vi "ProfilerTest.vi"() -> ()   [LabVIEW 2014] (continued)
"Velocity"=0.0}, {"Time"=2.6213203435596424, "Velocity"=0.0}, {"Time"=2.6213203435596424, "Velocity"=0.0}, {"Time"=2.6213203435596424, "Velocity"=0.0}, {"Time"=2.6213203435596424, "Velocity"=0.0}, {"Time"=2.6213203435596424, "Velocity"=0.0}, {"Time"=2.6213203435596424, "Velocity"=0.0}, {"Time"=2.6213203435596424, "Velocity"=0.0}, {"Time"=2.6213203435596424, "Velocity"=0.0}, {"Time"=2.6213203435596424, "Velocity"=0.0}, {"Time"=2.6213203435596424, "Velocity"=0.0}, {"Time"=2.6213203435596424, "Velocity"=0.0}, {"Time"=2.6213203435596424, "Velocity"=0.0}, {"Time"=2.6213203435596424, "Velocity"=0.0}, {"Time"=2.6213203435596424, "Velocity"=0.0}, {"Time"=2.6213203435596424, "Velocity"=0.0}, {"Time"=2.6213203435596424, "Velocity"=0.0}, {"Time"=2.6213203435596424, "Velocity"=0.0}, {"Time"=2.6213203435596424, "Velocity"=0.0}, {"Time"=2.6213203435596424, "Velocity"=0.0}, {"Time"=2.6213203435596424, "Velocity"=0.0}, {"Time"=2.6213203435596424, "Velocity"=0.0}, {"Time"=2.6213203435596424, "Velocity"=0.0}, {"Time"=2.6213203435596424, "Velocity"=0.0}, {"Time"=2.6213203435596424, "Velocity"=0.0}, {"Time"=2.6213203435596424, "Velocity"=0.0}, {"Time"=2.6213203435596424, "Velocity"=0.0}, {"Time"=2.6213203435596424, "Velocity"=0.0}, {"Time"=2.6213203435596424, "Velocity"=0.0}, {"Time"=2.6213203435596424, "Velocity"=0.0}, {"Time"=2.6213203435596424, "Velocity"=0.0}, {"Time"=2.6213203435596424, "Velocity"=0.0}, {"Time"=2.6213203435596424, "Velocity"=0.0}, {"Time"=2.6213203435596424, "Velocity"=0.0}, {"Time"=2.6213203435596424, "Velocity"=0.0}, {"Time"=2.6213203435596424, "Velocity"=0.0}, {"Time"=2.6213203435596424, "Velocity"=0.0}, {"Time"=2.6213203435596424, "Velocity"=0.0}, {"Time"=2.6213203435596424, "Velocity"=0.0}, {"Time"=2.6213203435596424, "Velocity"=0.0}, {"Time"=2.6213203435596424, "Velocity"=0.0}, {"Time"=2.6213203435596424, "Velocity"=0.0}, {"Time"=2.6213203435596424, "Velocity"=0.0}, {"Time"=2.6213203435596424, "Velocity"=0.0}, {"Time"=2.6213203435596424, "Velocity"=0.0}, {"Time"=2.6213203435596424, "Velocity"=0.0}, {"Time"=2.6213203435596424, "Velocity"=0.0}, {"Time"=2.6213203435596424, "Velocity"=0.0}, {"Time"=2.6213203435596424, "Velocity"=0.0}, {"Time"=2.6213203435596424, "Velocity"=0.0}, {"Time"=2.6213203435596424, "Velocity"=0.0}, {"Time"=2.6213203435596424, "Velocity"=0.0}, {"Time"=2.6213203435596424, "Velocity"=0.0}, {"Time"=2.6213203435596424, "Velocity"=0.0}, {"Time"=2.6213203435596424, "Velocity"=0.0}, {"Time"=2.6213203435596424, "Velocity"=0.0}, {"Time"=2.6213203435596424, "Velocity"=0.0}, {"Time"=2.6213203435596424, "Velocity"=0.0}, {"Time"=2.6213203435596424, "Velocity"=0.0}, {"Time"=2.6213203435596424, "Velocity"=0.0}, {"Time"=2.6213203435596424, "Velocity"=0.0}, {"Time"=2.6213203435596424, "Velocity"=0.0}, {"Time"=2.6213203435596424, "Velocity"=0.0}, {"Time"=2.6213203435596424, "Velocity"=0.0}, {"Time"=2.6213203435596424, "Velocity"=0.0}, {"Time"=2.6213203435596424, "Velocity"=0.0}, {"Time"=2.6213203435596424, "Velocity"=0.0}, {"Time"=2.6213203435596424, "Velocity"=0.0}, {"Time"=2.6213203435596424, "Velocity"=0.0}, {"Time"=2.6213203435596424, "Velocity"=0.0}, {"Time"=2.6213203435596424, "Velocity"=0.0}, {"Time"=2.6213203435596424, "Velocity"=0.0}, {"Time"=2.6213203435596424, "Velocity"=0.0}, {"Time"=2.6213203435596424, "Velocity"=0.0}, {"Time"=2.6213203435596424, "Velocity"=0.0}, {"Time"=2.6213203435596424, "Velocity"=0.0}, {"Time"=2.6213203435596424, "Velocity"=0.0}, {"Time"=2.6213203435596424, "Velocity"=0.0}, {"Time"=2.6213203435596424, "Velocity"=0.0}, {"Time"=2.6213203435596424, "Velocity"=0.0}, {"Time"=2.6213203435596424, "Velocity"=0.0}, {"Time"=2.6213203435596424, "Velocity"=0.0}, {"Time"=2.6213203435596424, "Velocity"=0.0}, {"Time"=2.6213203435596424, "Velocity"=0.0}, {"Time"=2.6213203435596424, "Velocity"=0.0}, {"Time"=2.6213203435596424, "Velocity"=0.0}, {"Time"=2.6213203435596424, "Velocity"=0.0}, {"Time"=2.6213203435596424, "Velocity"=0.0}, {"Time"=2.6213203435596424, "Velocity"=0.0}, {"Time"=2.6213203435596424, "Velocity"=0.0}, {"Time"=2.6213203435596424, "Velocity"=0.0}, {"Time"=2.6213203435596424, "Velocity"=0.0}, {"Time"=2.6213203435596424, "Velocity"=0.0}, {"Time"=2.6213203435596424, "Velocity"=0.0}, {"Time"=2.6213203435596424, "Velocity"=0.0}, {"Time"=2.6213203435596424, "Velocity"=0.0}, {"Time"=2.6213203435596424, "Velocity"=0.0}, {"Time"=3.179382300521122, "Velocity"=4.887545721840618e-11}, {"Time"=3.182363233638446, "Velocity"=0.004681906750662082}, {"Time"=3.1853442266817455, "Velocity"=0.018707612351687646}, {"Time"=3.1883251621540127, "Velocity"=0.04202122091463451}, {"Time"=3.1913058246256933, "Velocity"=0.0745275081352886}, {"Time"=3.194286771144685, "Velocity"=0.11610430676737167}, {"Time"=3.197267776397191, "Velocity"=0.1665859467999022}, {"Time"=3.2002486616525876, "Velocity"=0.22576990121215637}, {"Time"=3.2032293991934058, "Velocity"=0.2934208962549225}, {"Time"=3.2062103258323984, "Velocity"=0.36927975861350576}, {"Time"=3.2091913664944234, "Velocity"=0.45304642801194395}, {"Time"=3.212172348282649, "Velocity"=0.5443856615355546}, {"Time"=3.215153077010833, "Velocity"=0.6429298808695292}, {"Time"=3.2181341594868247, "Velocity"=0.7483105526778044}, {"Time"=3.2211147839090675, "Velocity"=0.860082815314104}, {"Time"=3.2240958267748936, "Velocity"=0.9778382408534675}, {"Time"=3.2270768318705443, "Velocity"=1.1010952117016748}, {"Time"=3.230057510835584, "Velocity"=1.2293544201841629}, {"Time"=3.2330383537653846, "Velocity"=1.3621303712216255}, {"Time"=3.2360195635020954, "Velocity"=1.4989092093095147}, {"Time"=3.239000371706686, "Velocity"=1.6391158529073055}, {"Time"=3.2419810306914276, "Velocity"=1.7822079438655614}, {"Time"=3.244961997160481, "Velocity"=1.9276428933754883}, {"Time"=3.2479428824398338, "Velocity"=2.074828061328674}, {"Time"=3.2509239694175522, "Velocity"=2.223196577850922}, {"Time"=3.2539048496185483, "Velocity"=2.372142581660095}, {"Time"=3.2568855225487265, "Velocity"=2.5210781729953533}, {"Time"=3.259866572626495, "Velocity"=2.6694447124446374}, {"Time"=3.262847615082643, "Velocity"=2.816637374438716}, {"Time"=3.2658284467512493, "Velocity"=2.962065373403272}, {"Time"=3.2688094528330196, "Velocity"=3.1051735478800238}, {"Time"=3.2717901011492847, "Velocity"=3.245371876903563}, {"Time"=3.2747710323978465, "Velocity"=3.38213728160929}, {"Time"=3.277752022417501, "Velocity"=3.514919121008004}, {"Time"=3.280732985554363, "Velocity"=3.643189467146226}, {"Time"=3.28371363478884, "Velocity"=3.7664305928082165}, {"Time"=3.2866947651209744, "Velocity"=3.8841884916299736}, {"Time"=3.2896756842649046, "Velocity"=3.99597034763491}, {"Time"=3.2926563514365763, "Velocity"=4.101334921685583}, {"Time"=3.2956374727404905, "Velocity"=4.199890633901769}, {"Time"=3.298618474379659, "Velocity"=4.291228403037818}, {"Time"=3.3015991540634593, "Velocity"=4.374983206384261}, {"Time"=3.304580116567556, "Velocity"=4.450841624260995}, {"Time"=3.30756083324709, "Velocity"=4.518490720524196}, {"Time"=3.3105420315563414, "Velocity"=4.577678998720427}, {"Time"=3.3135226724363, "Velocity"=4.628152609214704}, {"Time"=3.3165035991129286, "Velocity"=4.669727810948797}, {"Time"=3.319484620882282, "Velocity"=4.702236153213752}, {"Time"=3.322465509870618, "Velocity"=4.725547028669758}, {"Time"=3.3254465442327077, "Velocity"=4.739570548002267}, {"Time"=3.3284274714794138, "Velocity"=4.744249999882863}, {"Time"=3.3314083274309976, "Velocity"=4.739567811399099}, {"Time"=3.334389068020796, "Velocity"=4.725543407232389}, {"Time"=3.33736999085439, "Velocity"=4.702230421822115}, {"Time"=3.3403510145205813, "Velocity"=4.66972018065884}, {"Time"=3.343331845683909, "Velocity"=4.62814460377215}, {"Time"=3.3463127213565964, "Velocity"=4.577665140474008}, {"Time"=3.34929362108914, "Velocity"=4.518481048135488}, {"Time"=3.352274603067483, "Velocity"=4.450824289890841}, {"Time"=3.355255244905396, "Velocity"=4.3749725174933545}, {"Time"=3.358236366672093, "Velocity"=4.291203685185305}, {"Time"=3.3612170640143364, "Velocity"=4.19987352692686}, {"Time"=3.364197991665377, "Velocity"=4.101323178207656}, {"Time"=3.3671788958736792, "Velocity"=3.995949202532643}, {"Time"=3.370160002773235, "Velocity"=3.884158907986906}, {"Time"=3.373140697172389, "Velocity"=3.7664171646877844}, {"Time"=3.3761216862348933, "Velocity"=3.6431611066430656}, {"Time"=3.3791025119642133, "Velocity"=3.5148957069092033}, {"Time"=3.3820835823865347, "Velocity"=3.3821094679110097}, {"Time"=3.385064249730449, "Velocity"=3.245355564920387}, {"Time"=3.388045261129964, "Velocity"=3.10513959694406}, {"Time"=3.391026157018598, "Velocity"=2.962036133344201}, {"Time"=3.3940071550211357, "Velocity"=2.8165995512860045}, {"Time"=3.39698801785475, "Velocity"=2.6694154211857586}, {"Time"=3.399968948751446, "Velocity"=2.521054654482557}, {"Time"=3.4029497889706777, "Velocity"=2.372110652197633}, {"Time"=3.4059306352291676, "Velocity"=2.2231664051676723}, {"Time"=3.408911705934191, "Velocity"=2.07479887461014}, {"Time"=3.4118924656591023, "Velocity"=1.92762016228879}, {"Time"=3.414873470780533, "Velocity"=1.782183658015315}, {"Time"=3.4178541398265025, "Velocity"=1.6390915280380804}, {"Time"=3.4208351340590917, "Velocity"=1.4988767804771501}, {"Time"=3.4238160119268155, "Velocity"=1.362113826815595}, {"Time"=3.4267971471880583, "Velocity"=1.229325588696039}, {"Time"=3.4297779598240212, "Velocity"=1.1010617891916208}, {"Time"=3.4327588330093084, "Velocity"=0.9778115520210151}, {"Time"=3.435739589972038, "Velocity"=0.8600684112964558}, {"Time"=3.4387207610191526, "Velocity"=0.7482770016761722}, {"Time"=3.441701442053643, "Velocity"=0.6429121146564376}, {"Time"=3.4446823370875865, "Velocity"=0.544363817902734}, {"Time"=3.4476634251575002, "Velocity"=0.45302316196243675}, {"Time"=3.450644092312822, "Velocity"=0.3692685559349724}, {"Time"=3.4536252188140226, "Velocity"=0.29340600994766153}, {"Time"=3.456605936904525, "Velocity"=0.22575715851294909}, {"Time"=3.4595868836619856, "Velocity"=0.16657379756771834}, {"Time"=3.4625677175232754, "Velocity"=0.11609675641697091}, {"Time"=3.4655485614792525, "Velocity"=0.07452270710143796}, {"Time"=3.4685295280726667, "Velocity"=0.04201475404893379}, {"Time"=3.471510361955229, "Velocity"=0.018703923478933956}, {"Time"=3.474491413705976, "Velocity"=0.004679874386484596}, {"Time"=3.477472452833142, "Velocity"=1.0614160298802687e-10}, {"Time"=3.82842712474619, "Velocity"=0.0}, {"Time"=3.82842712474619, "Velocity"=0.0}, {"Time"=3.82842712474619, "Velocity"=0.0}, {"Time"=3.82842712474619, "Velocity"=0.0}, {"Time"=3.82842712474619, "Velocity"=0.0}, {"Time"=3.82842712474619, "Velocity"=0.0}, {"Time"=3.82842712474619, "Velocity"=0.0}, {"Time"=3.82842712474619, "Velocity"=0.0}, {"Time"=3.82842712474619, "Velocity"=0.0}, {"Time"=3.82842712474619, "Velocity"=0.0}, {"Time"=3.82842712474619, "Velocity"=0.0}, {"Time"=3.82842712474619, "Velocity"=0.0}, {"Time"=3.82842712474619, "Velocity"=0.0}, {"Time"=3.82842712474619, "Velocity"=0.0}, {"Time"=3.82842712474619, "Velocity"=0.0}, {"Time"=3.82842712474619, "Velocity"=0.0}, {"Time"=3.82842712474619, "Velocity"=0.0}, {"Time"=3.82842712474619, "Velocity"=0.0}, {"Time"=3.82842712474619, "Velocity"=0.0}, {"Time"=3.82842712474619, "Velocity"=0.0}, {"Time"=3.82842712474619, "Velocity"=0.0}, {"Time"=3.82842712474619, "Velocity"=0.0}, {"Time"=3.82842712474619, "Velocity"=0.0}, {"Time"=3.82842712474619, "Velocity"=0.0}, {"Time"=3.82842712474619, "Velocity"=0.0}, {"Time"=3.82842712474619, "Velocity"=0.0}, {"Time"=3.82842712474619, "Velocity"=0.0}, {"Time"=3.82842712474619, "Velocity"=0.0}, {"Time"=3.82842712474619, "Velocity"=0.0}, {"Time"=3.82842712474619, "Velocity"=0.0}, {"Time"=3.82842712474619, "Velocity"=0.0}, {"Time"=3.82842712474619, "Velocity"=0.0}, {"Time"=3.82842712474619, "Velocity"=0.0}, {"Time"=3.82842712474619, "Velocity"=0.0}, {"Time"=3.82842712474619, "Velocity"=0.0}, {"Time"=3.82842712474619, "Velocity"=0.0}, {"Time"=3.82842712474619, "Velocity"=0.0}, {"Time"=3.82842712474619, "Velocity"=0.0}, {"Time"=3.82842712474619, "Velocity"=0.0}, {"Time"=3.82842712474619, "Velocity"=0.0}, {"Time"=3.82842712474619, "Velocity"=0.0}, {"Time"=3.82842712474619, "Velocity"=0.0}, {"Time"=3.82842712474619, "Velocity"=0.0}, {"Time"=3.82842712474619, "Velocity"=0.0}, {"Time"=3.82842712474619, "Velocity"=0.0}, {"Time"=3.82842712474619, "Velocity"=0.0}, {"Time"=3.82842712474619, "Velocity"=0.0}, {"Time"=3.82842712474619, "Velocity"=0.0}, {"Time"=3.82842712474619, "Velocity"=0.0}, {"Time"=3.82842712474619, "Velocity"=0.0}, {"Time"=3.82842712474619, "Velocity"=0.0}, {"Time"=3.82842712474619, "Velocity"=0.0}, {"Time"=3.82842712474619, "Velocity"=0.0}, {"Time"=3.82842712474619, "Velocity"=0.0}, {"Time"=3.82842712474619, "Velocity"=0.0}, {"Time"=3.82842712474619, "Velocity"=0.0}, {"Time"=3.82842712474619, "Velocity"=0.0}, {"Time"=3.82842712474619, "Velocity"=0.0}, {"Time"=3.82842712474619, "Velocity"=0.0}, {"Time"=3.82842712474619, "Velocity"=0.0}, {"Time"=3.82842712474619, "Velocity"=0.0}, {"Time"=3.82842712474619, "Velocity"=0.0}, {"Time"=3.82842712474619, "Velocity"=0.0}, {"Time"=3.82842712474619, "Velocity"=0.0}, {"Time"=3.82842712474619, "Velocity"=0.0}, {"Time"=3.82842712474619, "Velocity"=0.0}, {"Time"=3.82842712474619, "Velocity"=0.0}, {"Time"=3.82842712474619, "Velocity"=0.0}, {"Time"=3.82842712474619, "Velocity"=0.0}, {"Time"=3.82842712474619, "Velocity"=0.0}, {"Time"=3.82842712474619, "Velocity"=0.0}, {"Time"=3.82842712474619, "Velocity"=0.0}, {"Time"=3.82842712474619, "Velocity"=0.0}, {"Time"=3.82842712474619, "Velocity"=0.0}, {"Time"=3.82842712474619, "Velocity"=0.0}, {"Time"=3.82842712474619, "Velocity"=0.0}, {"Time"=3.82842712474619, "Velocity"=0.0}, {"Time"=3.82842712474619, "Velocity"=0.0}, {"Time"=3.82842712474619, "Velocity"=0.0}, {"Time"=3.82842712474619, "Velocity"=0.0}, {"Time"=3.82842712474619, "Velocity"=0.0}, {"Time"=3.82842712474619, "Velocity"=0.0}, {"Time"=3.82842712474619, "Velocity"=0.0}, {"Time"=3.82842712474619, "Velocity"=0.0}, {"Time"=3.82842712474619, "Velocity"=0.0}, {"Time"=3.82842712474619, "Velocity"=0.0}, {"Time"=3.82842712474619, "Velocity"=0.0}, {"Time"=3.82842712474619, "Velocity"=0.0}, {"Time"=3.82842712474619, "Velocity"=0.0}, {"Time"=3.82842712474619, "Velocity"=0.0}, {"Time"=3.82842712474619, "Velocity"=0.0}, {"Time"=3.82842712474619, "Velocity"=0.0}, {"Time"=3.82842712474619, "Velocity"=0.0}, {"Time"=3.82842712474619, "Velocity"=0.0}, {"Time"=3.82842712474619, "Velocity"=0.0}, {"Time"=3.82842712474619, "Velocity"=0.0}, {"Time"=3.82842712474619, "Velocity"=0.0}, {"Time"=3.82842712474619, "Velocity"=0.0}, {"Time"=3.82842712474619, "Velocity"=0.0}, {"Time"=3.82842712474619, "Velocity"=0.0}, {"Time"=3.82842712474619, "Velocity"=0.0}]}, ...(2 in all)]
  out "XY Graph":T5(graph)=[{"XY Graph"=[{"X"=0.0, "Y"=0.0}, {"X"=0.0, "Y"=0.5}, {"X"=0.5, "Y"=1.0}, {"X"=1.0, "Y"=0.5}, {"X"=0.5, "Y"=0.0}, {"X"=0.0, "Y"=0.5}]}, {"XY Graph"=[{"X"=0.0, "Y"=0.029735763271532455}, {"X"=0.0, "Y"=0.03498550646188265}, {"X"=0.0, "Y"=0.04073166444158789}, {"X"=0.0, "Y"=0.046965098069385154}, {"X"=0.0, "Y"=0.053670825690082614}, {"X"=0.0, "Y"=0.06082839203263177}, {"X"=0.0, "Y"=0.06841237188678788}, {"X"=0.0, "Y"=0.0763929961561675}, {"X"=0.0, "Y"=0.0847368848721995}, {"X"=0.0, "Y"=0.09340786911973305}, {"X"=0.0, "Y"=0.10236788163576621}, {"X"=0.0, "Y"=0.11157789415179944}, {"X"=0.0, "Y"=0.12099887839933296}, {"X"=0.0, "Y"=0.1305927671153649}, {"X"=0.0, "Y"=0.14032339138474453}, {"X"=0.0, "Y"=0.15015737123890066}, {"X"=0.0, "Y"=0.16006493758144982}, {"X"=0.0, "Y"=0.1700206652021473}, {"X"=0.0, "Y"=0.18000409882994453}, {"X"=0.0, "Y"=0.19000025680964983}, {"X"=0.0, "Y"=0.20000000000000004}, {"X"=0.0, "Y"=0.21000000000000005}, {"X"=0.0, "Y"=0.22000000000000006}, {"X"=0.0, "Y"=0.23000000000000007}, {"X"=0.0, "Y"=0.24000000000000007}, {"X"=0.0, "Y"=0.25000000000000006}, {"X"=0.0, "Y"=0.26000000000000006}, {"X"=0.0, "Y"=0.2700000000000001}, {"X"=0.0, "Y"=0.2800000000000001}, {"X"=0.0, "Y"=0.2900000000000001}, {"X"=0.0, "Y"=0.3000000000000001}, {"X"=0.0, "Y"=0.3100000000000001}, {"X"=0.0, "Y"=0.3200000000000001}, {"X"=0.0, "Y"=0.3300000000000001}, {"X"=0.0, "Y"=0.34000000000000014}, {"X"=3.652435472123461e-11, "Y"=0.35000000000000014}, {"X"=2.9356280516375233e-07, "Y"=0.36000000000000015}, {"X"=5.746236574666157e-06, "Y"=0.37000000000000016}, {"X"=3.086411351601627e-05, "Y"=0.38000000000000017}, {"X"=9.978288886692112e-05, "Y"=0.3900000000000002}, {"X"=0.00024519954102164955, "Y"=0.3999999811877839}, {"X"=0.0005069250135350944, "Y"=0.40999991604546854}, {"X"=0.00093012200045119, "Y"=0.41999565182389387}, {"X"=0.0015633058386469356, "Y"=0.42996991190655165}, {"X"=0.002456196996851569, "Y"=0.43989147316712146}, {"X"=0.0036575202200111994, "Y"=0.44971848515533863}, {"X"=0.005212847748947858, "Y"=0.45940291902442193}, {"X"=0.007162582084287682, "Y"=0.4688956732552045}, {"X"=0.009540167586764372, "Y"=0.47815179341109415}, {"X"=0.012370610076658345, "Y"=0.4871352510359044}, {"X"=0.015669369961679704, "Y"=0.4958227736720711}, {"X"=0.019441677888523835, "Y"=0.5042063188477698}, {"X"=0.02368230321049537, "Y"=0.5122939290348251}, {"X"=0.02837578551988419, "Y"=0.5201088766908009}, {"X"=0.033497118996409864, "Y"=0.5276871902718838}, {"X"=0.03901285927933871, "Y"=0.535073824214666}, {"X"=0.04488260386804458, "Y"=0.5423178800383143}, {"X"=0.051060780521705436, "Y"=0.5494673865896099}, {"X"=0.057498664495375204, "Y"=0.5565641943188177}, {"X"=0.06414653532032459, "Y"=0.5636395263522579}, {"X"=0.07095587765967663, "Y"=0.5707106781186551}, {"X"=0.0778815288193874, "Y"=0.5777817459305206}, {"X"=0.08488367785590198, "Y"=0.5848528137423861}, {"X"=0.09192962779082611, "Y"=0.5919238815542516}, {"X"=0.09899524292892209, "Y"=0.598994949366117}, {"X"=0.10606601717798247, "Y"=0.6060660171779825}, {"X"=0.11313708498984798, "Y"=0.613137084989848}, {"X"=0.12020815280171349, "Y"=0.6202081528017135}, {"X"=0.127279220613579, "Y"=0.6272792206135789}, {"X"=0.1343502884254444, "Y"=0.6343502884254444}, {"X"=0.1414213562373099, "Y"=0.6414213562373099}, {"X"=0.1484924240491754, "Y"=0.6484924240491754}, {"X"=0.1555634918610409, "Y"=0.6555634918610409}, {"X"=0.1626345596729063, "Y"=0.6626345596729063}, {"X"=0.1697056274847718, "Y"=0.6697056274847718}, {"X"=0.1767766952966373, "Y"=0.6767766952966373}, {"X"=0.18384776310850282, "Y"=0.6838477631085028}, {"X"=0.1909188309203682, "Y"=0.6909188309203682}, {"X"=0.19798989873223372, "Y"=0.6979898987322337}, {"X"=0.20506096654409922, "Y"=0.7050609665440992}, {"X"=0.21213203435596473, "Y"=0.7121320343559647}, {"X"=0.21920310216783023, "Y"=0.7192031021678302}, {"X"=0.22627416997969563, "Y"=0.7262741699796956}, {"X"=0.23334523779156113, "Y"=0.7333452377915611}, {"X"=0.24041630560342664, "Y"=0.7404163056034266}, {"X"=0.24748737341529214, "Y"=0.7474873734152921}, {"X"=0.25455844122715754, "Y"=0.7545584412271575}, {"X"=0.26162950903902304, "Y"=0.761629509039023}, {"X"=0.26870057685088855, "Y"=0.7687005768508886}, {"X"=0.27577164466275406, "Y"=0.7757716446627541}, {"X"=0.28284271247461956, "Y"=0.7828427124746196}, {"X"=0.28991378028648496, "Y"=0.789913780286485}, {"X"=0.29698484809835046, "Y"=0.7969848438501712}, {"X"=0.30405591591021597, "Y"=0.8040559020012281}, {"X"=0.3111269837220814, "Y"=0.8111261965564864}, {"X"=0.3181980515339469, "Y"=0.818192429217553}, {"X"=0.3252691193458124, "Y"=0.8252482706643375}, {"X"=0.3323401871576779, "Y"=0.8322844385596649}, {"X"=0.3394112549695434, "Y"=0.8392888119478362}, {"X"=0.34648232278140884, "Y"=0.8462465806372527}, {"X"=0.35355339059327434, "Y"=0.8531404277260638}, {"X"=0.3606244584051398, "Y"=0.8599507430213329}, {"X"=0.3676955262170053, "Y"=0.866655864721471}, {"X"=0.37476659402887075, "Y"=0.8732323463833699}, {"X"=0.38183766184073625, "Y"=0.879655245884038}, {"X"=0.3889087296526017, "Y"=0.8858984328154871}, {"X"=0.3959797974644672, "Y"=0.8919349105244312}, {"X"=0.4030508652763327, "Y"=0.897737148827876}, {"X"=0.41012193308819817, "Y"=0.903277423304103}, {"X"=0.41719300090006367, "Y"=0.9085281569775152}, {"X"=0.4242640687119291, "Y"=0.9134622601863093}, {"X"=0.4313351365237946, "Y"=0.9180534644443316}, {"X"=0.4384062043356601, "Y"=0.9222766461824984}, {"X"=0.4454772721475256, "Y"=0.9261081363798823}, {"X"=0.45254833995939103, "Y"=0.9295260122684721}, {"X"=0.45961940777125654, "Y"=0.9325103675165388}, {"X"=0.46669047558312204, "Y"=0.9350435575607832}, {"X"=0.4737615433949875, "Y"=0.9371104170637072}, {"X"=0.480832611206853, "Y"=0.9386984468161961}, {"X"=0.48790367901871845, "Y"=0.9397979677818618}, {"X"=0.49497474683058396, "Y"=0.9404022403846553}, {"X"=0.5020458146424494, "Y"=0.9405075475696062}, {"X"=0.5091168824543149, "Y"=0.9401132406130259}, {"X"=0.5161879502661804, "Y"=0.9392217471175893}, {"X"=0.5232590180780459, "Y"=0.9378385410937662}, {"X"=0.5303300858899114, "Y"=0.935972075496324}, {"X"=0.5374011537017769, "Y"=0.9336336780473475}, {"X"=0.5444722215136424, "Y"=0.9308374116296854}, {"X"=0.5515432893255078, "Y"=0.9275999009713787}, {"X"=0.5586143571373733, "Y"=0.9239401277570739}, {"X"=0.5656854249492388, "Y"=0.9198791966915286}, {"X"=0.5727564927611042, "Y"=0.9154400753983241}, {"X"=0.5798275605729697, "Y"=0.9106473113593563}, {"X"=0.5868986283848352, "Y"=0.9055267293836362}, {"X"=0.5939696961967007, "Y"=0.9001051133338924}, {"X"=0.6010407640085662, "Y"=0.8944098760334825}, {"X"=0.6081118318204316, "Y"=0.8884687214217868}, {"X"=0.6151828996322971, "Y"=0.8823093031217938}, {"X"=0.6222539674441626, "Y"=0.8759588836278015}, {"X"=0.6293250352560281, "Y"=0.8694439983135156}, {"X"=0.6363961030678935, "Y"=0.8627901284014213}, {"X"=0.643467170879759, "Y"=0.8560213869238579}, {"X"=0.6505382386916245, "Y"=0.8491602215461183}, {"X"=0.65760930650349, "Y"=0.8422271379140758}, {"X"=0.6646803743153555, "Y"=0.8352404469358942}, {"X"=0.6717514421272209, "Y"=0.8282160391124034}, {"X"=0.6788225099390864, "Y"=0.8211671886973672}, {"X"=0.6858935777509519, "Y"=0.814104390101236}, {"X"=0.6929646455628174, "Y"=0.8070352285545984}, {"X"=0.7000357133746828, "Y"=0.799964286625317}, {"X"=0.7071067811865483, "Y"=0.7928932188134515}, {"X"=0.7141778489984139, "Y"=0.785822151001586}, {"X"=0.7212489168102794, "Y"=0.7787510831897205}, {"X"=0.7283199846221449, "Y"=0.7716800153778551}, {"X"=0.7353910524340103, "Y"=0.7646089475659896}, {"X"=0.7424621202458758, "Y"=0.7575378797541241}, {"X"=0.7495331880577413, "Y"=0.7504668119422586}, {"X"=0.7566042558696068, "Y"=0.7433957441303932}, {"X"=0.7636753236814722, "Y"=0.7363246763185277}, {"X"=0.7707463914933377, "Y"=0.7292536085066622}, {"X"=0.7778174593052032, "Y"=0.7221825406947967}, {"X"=0.7848885271170687, "Y"=0.7151114728829312}, {"X"=0.7919595949289342, "Y"=0.7080404050710658}, {"X"=0.7990306626954164, "Y"=0.7009693372592003}, {"X"=0.8061016593202558, "Y"=0.6938982694473348}, {"X"=0.8131712527865763, "Y"=0.6868272016354694}, {"X"=0.8202352620120484, "Y"=0.6797561338236039}, {"X"=0.827286493654544, "Y"=0.6726850660117384}, {"X"=0.8343148307652385, "Y"=0.6656139981998729}, {"X"=0.8413073574731994, "Y"=0.6585429303880075}, {"X"=0.8482485181648056, "Y"=0.651471862576142}, {"X"=0.8551203091962207, "Y"=0.6444007947642765}, {"X"=0.8619025007761909, "Y"=0.637329726952411}, {"X"=0.8685728862846124, "Y"=0.6302586591405455}, {"X"=0.8751075559541842, "Y"=0.6231875913286801}, {"X"=0.8814811915422052, "Y"=0.6161165235168146}, {"X"=0.8876673783608819, "Y"=0.6090454557049491}, {"X"=0.893638930820585, "Y"=0.6019743878930836}, {"X"=0.8993682274739522, "Y"=0.5949033200812182}, {"X"=0.9048275514316437, "Y"=0.5878322522693527}, {"X"=0.909989431954358, "Y"=0.5807611844574871}, {"X"=0.9148269830112109, "Y"=0.5736901166456216}, {"X"=0.9193142346319794, "Y"=0.5666190488337561}, {"X"=0.923426452969513, "Y"=0.5595479810218907}, {"X"=0.9271404451277594, "Y"=0.5524769132100252}, {"X"=0.930434844998606, "Y"=0.5454058453981597}, {"X"=0.9332903765847869, "Y"=0.5383347775862942}, {"X"=0.9356900915635825, "Y"=0.5312637097744288}, {"X"=0.9376195781634938, "Y"=0.5241926419625633}, {"X"=0.939067138779631, "Y"=0.5171215741506978}, {"X"=0.9400239341388239, "Y"=0.5100505063388323}, {"X"=0.9404840922377169, "Y"=0.5029794385269668}, {"X"=0.9404447807112605, "Y"=0.4959083707151014}, {"X"=0.9399062417397042, "Y"=0.4888373029032359}, {"X"=0.9388717890638885, "Y"=0.4817662350913704}, {"X"=0.9373477671456181, "Y"=0.4746951672795049}, {"X"=0.9353434729764385, "Y"=0.4676240994676395}, {"X"=0.93287104149847, "Y"=0.460553031655774}, {"X"=0.9299452960494095, "Y"=0.4534819638439085}, {"X"=0.9265835656748664, "Y"=0.446410896032043}, {"X"=0.9228054715595341, "Y"=0.4393398282201777}, {"X"=0.9186326852092874, "Y"=0.43226876040831236}, {"X"=0.9140886613644543, "Y"=0.425197692596447}, {"X"=0.9091983489359196, "Y"=0.41812662478458174}, {"X"=0.9039878835265829, "Y"=0.4110555569727164}, {"X"=0.8984842653276365, "Y"=0.40398448916085106}, {"X"=0.8927150263593732, "Y"=0.3969134213489858}, {"X"=0.8867078911575582, "Y"=0.3898423535371204}, {"X"=0.8804904350871787, "Y"=0.3827712857252551}, {"X"=0.8740897444946213, "Y"=0.37570021791338976}, {"X"=0.867532082886675, "Y"=0.3686291501015244}, {"X"=0.8608425672504805, "Y"=0.36155808228965913}, {"X"=0.8540448585035596, "Y"=0.3544870144777938}, {"X"=0.8471608698889264, "Y"=0.34741594666592845}, {"X"=0.8402104969091082, "Y"=0.34034487885406317}, {"X"=0.8332113721274628, "Y"=0.33327381104219783}, {"X"=0.8261786478586969, "Y"=0.3262027432303325}, {"X"=0.8191248094267816, "Y"=0.3191316754184672}, {"X"=0.8120595212917334, "Y"=0.31206060760660187}, {"X"=0.8049895079416476, "Y"=0.30498953979473653}, {"X"=0.7979184719828709, "Y"=0.2979184719828712}, {"X"=0.7908474041710055, "Y"=0.29084740417100585}, {"X"=0.7837763363591402, "Y"=0.28377633635914057}, {"X"=0.776705268547275, "Y"=0.27670526854727523}, {"X"=0.7696342007354096, "Y"=0.2696342007354099}, {"X"=0.7625631329235443, "Y"=0.2625631329235446}, {"X"=0.755492065111679, "Y"=0.25549206511167927}, {"X"=0.7484209972998136, "Y"=0.24842099729981393}, {"X"=0.7413499294879483, "Y"=0.24134992948794862}, {"X"=0.7342788616760829, "Y"=0.2342788616760833}, {"X"=0.7272077938642176, "Y"=0.22720779386421797}, {"X"=0.7201367260523523, "Y"=0.22013672605235263}, {"X"=0.713065658240487, "Y"=0.21306565824048732}, {"X"=0.7059945904286217, "Y"=0.20599465678890416}, {"X"=0.6989235226167564, "Y"=0.1989235226857829}, {"X"=0.691852454804891, "Y"=0.1918526812007721}, {"X"=0.6847813869930257, "Y"=0.18478413913976788}, {"X"=0.6777103191811604, "Y"=0.1777229560516226}, {"X"=0.670639251369295, "Y"=0.1706771818726091}, {"X"=0.6635681835574297, "Y"=0.16365775771637187}, {"X"=0.6564971157455645, "Y"=0.156678381032062}, {"X"=0.6494260479336991, "Y"=0.14975533679249164}, {"X"=0.6423549801218338, "Y"=0.14290729679279982}, {"X"=0.6352839123099684, "Y"=0.13615508953313904}, {"X"=0.6282128444981031, "Y"=0.12952144352142347}, {"X"=0.6211417766862378, "Y"=0.12303070715975975}, {"X"=0.6140707088743724, "Y"=0.11670854866677154}, {"X"=0.6069996410625071, "Y"=0.11058163973407363}, {"X"=0.5999285732506419, "Y"=0.10467732681561628}, {"X"=0.5928575054387765, "Y"=0.09902329410103804}, {"X"=0.5857864376269112, "Y"=0.09364722232665312}, {"X"=0.5787153698150459, "Y"=0.08857644762899884}, {"X"=0.5716443020031805, "Y"=0.08383762464534342}, {"X"=0.5645732341913152, "Y"=0.07945639801321384}, {"X"=0.5575021663794499, "Y"=0.07545708631749096}, {"X"=0.5504310985675845, "Y"=0.07186238238021145}, {"X"=0.5433600307557193, "Y"=0.0686930735868029}, {"X"=0.536288962943854, "Y"=0.06596778569554357}, {"X"=0.5292178951319886, "Y"=0.0637027532876219}, {"X"=0.5221468273201233, "Y"=0.06191161968684569}, {"X"=0.515075759508258, "Y"=0.06060526881485456}, {"X"=0.5080046916963926, "Y"=0.059791691054108226}, {"X"=0.5009336238845273, "Y"=0.05947588477179813}, {"X"=0.493862556072662, "Y"=0.05965979471833446}, {"X"=0.4867914882607967, "Y"=0.06034228805960601}, {"X"=0.4797204204489314, "Y"=0.061519168338398045}, {"X"=0.47264935263706603, "Y"=0.06318322719290465}, {"X"=0.4655782848252007, "Y"=0.06532433319493813}, {"X"=0.4585072170133354, "Y"=0.06792955671296586}, {"X"=0.45143614920147007, "Y"=0.07098332926111983}, {"X"=0.44436508138960473, "Y"=0.07446763537031173}, {"X"=0.43729401357773945, "Y"=0.07836223461676894}, {"X"=0.4302229457658741, "Y"=0.08264491107164071}, {"X"=0.42315187795400877, "Y"=0.08729174709737533}, {"X"=0.41608081014214343, "Y"=0.09227741811651229}, {"X"=0.40900974233027815, "Y"=0.09757550472006164}, {"X"=0.4019386745184128, "Y"=0.10315881826894656}, {"X"=0.39486760670654747, "Y"=0.10899973597568793}, {"X"=0.38779653889468213, "Y"=0.11507054133667717}, {"X"=0.38072547108281685, "Y"=0.12134376571943582}, {"X"=0.3736544032709515, "Y"=0.1277925268950321}, {"X"=0.36658333545908617, "Y"=0.1343908603434663}, {"X"=0.3595122676472209, "Y"=0.1411140392489125}, {"X"=0.35244119983535555, "Y"=0.14793887924108806}, {"X"=0.3453701320234902, "Y"=0.15484402412702025}, {"X"=0.33829906421162487, "Y"=0.16181020909175664}, {"X"=0.33122799639975953, "Y"=0.16882049812424904}, {"X"=0.32415692858789424, "Y"=0.17586049274229573}, {"X"=0.3170858607760289, "Y"=0.182918509444148}, {"X"=0.31001479296416357, "Y"=0.18998572369980893}, {"X"=0.3029437251522983, "Y"=0.19705627870742862}, {"X"=0.29587265734043294, "Y"=0.2041273426595669}, {"X"=0.2888015895285676, "Y"=0.21119841047143223}, {"X"=0.28173052171670226, "Y"=0.21826947828329754}, {"X"=0.274659453904837, "Y"=0.22534054609516285}, {"X"=0.26758838609297164, "Y"=0.2324116139070282}, {"X"=0.2605173182811063, "Y"=0.2394826817188935}, {"X"=0.25344625046924096, "Y"=0.24655374953075884}, {"X"=0.24637518265737568, "Y"=0.2536247960999044}, {"X"=0.23930411484551034, "Y"=0.26069588444560143}, {"X"=0.232233047033645, "Y"=0.26776670163736305}, {"X"=0.2251619792217797, "Y"=0.27483555885382616}, {"X"=0.21809091140991438, "Y"=0.2818986686541452}, {"X"=0.21101984359804904, "Y"=0.2889501770228091}, {"X"=0.20394877578618373, "Y"=0.2959822128993532}, {"X"=0.19687770797431842, "Y"=0.30298495477390514}, {"X"=0.18980664016245308, "Y"=0.30994671378511207}, {"X"=0.18273557235058774, "Y"=0.3168540326173743}, {"X"=0.17566450453872243, "Y"=0.32369179936063314}, {"X"=0.16859343672685712, "Y"=0.3304433753693684}, {"X"=0.16152236891499178, "Y"=0.3370907360390143}, {"X"=0.15445130110312644, "Y"=0.343614623308711}, {"X"=0.14738023329126113, "Y"=0.3499947086000957}, {"X"=0.14030916547939581, "Y"=0.3562097648135383}, {"X"=0.13323809766753048, "Y"=0.3622378459265951}, {"X"=0.12616702985566516, "Y"=0.3680564726751312}, {"X"=0.11909596204379984, "Y"=0.3736428227461003}, {"X"=0.11202523403573622, "Y"=0.3789739238727948}, {"X"=0.10495382642646973, "Y"=0.38402684819882693}, {"X"=0.09788331581713505, "Y"=0.38877890626636086}, {"X"=0.09081957638444334, "Y"=0.3932078389873016}, {"X"=0.08377868269332125, "Y"=0.39729200597320646}, {"X"=0.0767861981630556, "Y"=0.4010105686304961}, {"X"=0.0698760435132908, "Y"=0.40434366647183295}, {"X"=0.06308899527764128, "Y"=0.40727258515192766}, {"X"=0.05647088084758199, "Y"=0.40977991480605547}, {"X"=0.05007054994224022, "Y"=0.4118496973516119}, {"X"=0.04393771229612516, "Y"=0.4134675615064143}, {"X"=0.038120737278638225, "Y"=0.4146208443813882}, {"X"=0.03266451284428114, "Y"=0.4152986986188634}, {"X"=0.02760845858623022, "Y"=0.4154921841700049}, {"X"=0.022984780844624783, "Y"=0.4151943439348656}, {"X"=0.018817047106467102, "Y"=0.4144002626250866}, {"X"=0.015119142800722948, "Y"=0.4131071083512168}, {"X"=0.011894656665648928, "Y"=0.41131415658279125}, {"X"=0.009136721894802802, "Y"=0.40902279627844584}, {"X"=0.006828320093342513, "Y"=0.4062365181342021}, {"X"=0.004943034590115844, "Y"=0.4029608850493518}, {"X"=0.003446219760497679, "Y"=0.3992034850598246}, {"X"=0.002296534600391878, "Y"=0.3949738671372581}, {"X"=0.0014477726683890524, "Y"=0.39028346039696515}, {"X"=0.0008509073944608092, "Y"=0.38514547739836236}, {"X"=0.00045626222046078746, "Y"=0.3795748023560175}, {"X"=0.00021570951207672273, "Y"=0.3735878652071398}, {"X"=8.480090832024834e-05, "Y"=0.3672025026010065}, {"X"=2.473480953069096e-05, "Y"=0.36043780698646405}, {"X"=4.073913863492096e-06, "Y"=0.35331396507434965}, {"X"=1.3677623388053117e-07, "Y"=0.34585208704156944}, {"X"=1.3677623388053117e-07, "Y"=0.33807402792190533}, {"X"=1.3677623388053117e-07, "Y"=0.3300022026947312}, {"X"=1.3677623388053117e-07, "Y"=0.3216593966361336}, {"X"=1.3677623388053117e-07, "Y"=0.31306857253702436}, {"X"=1.3677623388053117e-07, "Y"=0.3042526764193328}, {"X"=1.3677623388053117e-07, "Y"=0.2952344433940779}, {"X"=1.3677623388053117e-07, "Y"=0.2860362053039169}, {"X"=1.3677623388053117e-07, "Y"=0.27667970177767115}, {"X"=1.3677623388053117e-07, "Y"=0.26718589629546097}, {"X"=1.3677623388053117e-07, "Y"=0.25757479882068623}, {"X"=1.3677623388053117e-07, "Y"=0.24786529649953135}, {"X"=1.3677623388053117e-07, "Y"=0.2380749938604127}, {"X"=1.3677623388053117e-07, "Y"=0.22822006386541183}, {"X"=1.3677623388053117e-07, "Y"=0.218315111073918}, {"X"=1.3677623388053117e-07, "Y"=0.20837304807622908}, {"X"=1.3677623388053117e-07, "Y"=0.19840498624257943}, {"X"=1.3677623388053117e-07, "Y"=0.18842014171195087}, {"X"=1.3677623388053117e-07, "Y"=0.17842575741607147}, {"X"=1.3677623388053117e-07, "Y"=0.16842704179834855}, {"X"=1.3677623388053117e-07, "Y"=0.16842704179834855}, {"X"=1.3677623388053117e-07, "Y"=0.16842704179834855}, {"X"=1.3677623388053117e-07, "Y"=0.16842704179834855}, {"X"=1.3677623388053117e-07, "Y"=0.16842704179834855}, {"X"=1.3677623388053117e-07, "Y"=0.16842704179834855}, {"X"=1.3677623388053117e-07, "Y"=0.16842704179834855}, {"X"=1.3677623388053117e-07, "Y"=0.16842704179834855}, {"X"=1.3677623388053117e-07, "Y"=0.16842704179834855}, {"X"=1.3677623388053117e-07, "Y"=0.16842704179834855}, {"X"=1.3677623388053117e-07, "Y"=0.16842704179834855}, {"X"=1.3677623388053117e-07, "Y"=0.16842704179834855}, {"X"=1.3677623388053117e-07, "Y"=0.16842704179834855}, {"X"=1.3677623388053117e-07, "Y"=0.16842704179834855}, {"X"=1.3677623388053117e-07, "Y"=0.16842704179834855}, {"X"=1.3677623388053117e-07, "Y"=0.16842704179834855}, {"X"=1.3677623388053117e-07, "Y"=0.16842704179834855}, {"X"=1.3677623388053117e-07, "Y"=0.16842704179834855}, {"X"=1.3677623388053117e-07, "Y"=0.16842704179834855}, {"X"=1.3677623388053117e-07, "Y"=0.16842704179834855}, {"X"=1.3677623388053117e-07, "Y"=0.16842704179834855}, {"X"=1.3677623388053117e-07, "Y"=0.16842704179834855}, {"X"=1.3677623388053117e-07, "Y"=0.16842704179834855}, {"X"=1.3677623388053117e-07, "Y"=0.16842704179834855}, {"X"=1.3677623388053117e-07, "Y"=0.16842704179834855}, {"X"=1.3677623388053117e-07, "Y"=0.16842704179834855}, {"X"=1.3677623388053117e-07, "Y"=0.16842704179834855}, {"X"=1.3677623388053117e-07, "Y"=0.16842704179834855}, {"X"=1.3677623388053117e-07, "Y"=0.16842704179834855}, {"X"=1.3677623388053117e-07, "Y"=0.16842704179834855}, {"X"=1.3677623388053117e-07, "Y"=0.16842704179834855}, 
